vi "_createKafkaEvents.vi"(0 "Payload":string[](array[string]), 3 "error in (no error)":errorcluster, 4 "Debug":bool) -> (7 "Kafka Events":T1[](array[typedef]), 10 "error out":errorcluster)   [LabVIEW 2019]
uses:
  KafkaLVLib/API/KafkaConsumerEvent.ctl
  1f099e04-d0a3-4231-929c-9bf0d6f2adbc.vi
  <vilib>/JDP Science/JSONtext/String Subset.vi
  <vilib>/JDP Science/JSONtext/Parsing/Parse Full Path or Item Name.vi
  <vilib>/JDP Science/JSONtext/Next JSON Value.vi
  <vilib>/JDP Science/JSONtext/support/Error Cluster From Code.vi
  <vilib>/JDP Science/JSONtext/Offset/Find Item Locations by Path.vi
  <vilib>/JDP Science/JSONtext/JSON text to Variant.vi
  <vilib>/JDP Science/JSONtext/JSONtext.lvlib
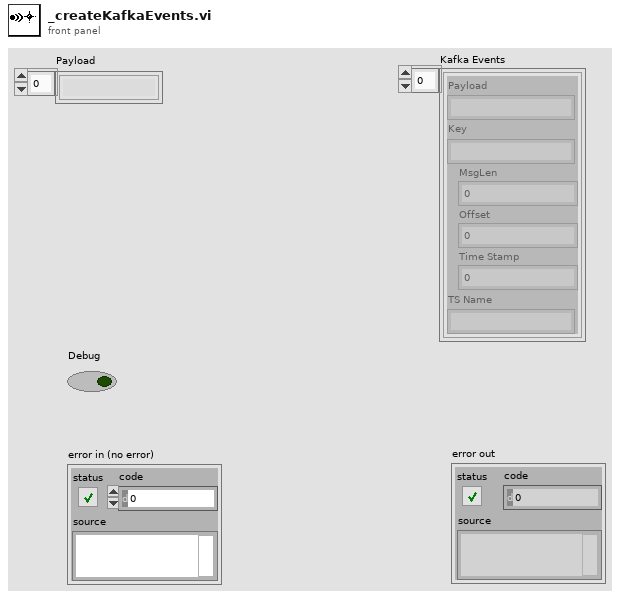
[diagram p1: front panel]
types:
  T1 = typedef "KafkaConsumerEvent.ctl" = cluster{"Payload":string, "Key":string, "MsgLen":u64, "Offset":i64, "Time Stamp":i64, "TS Name":string}
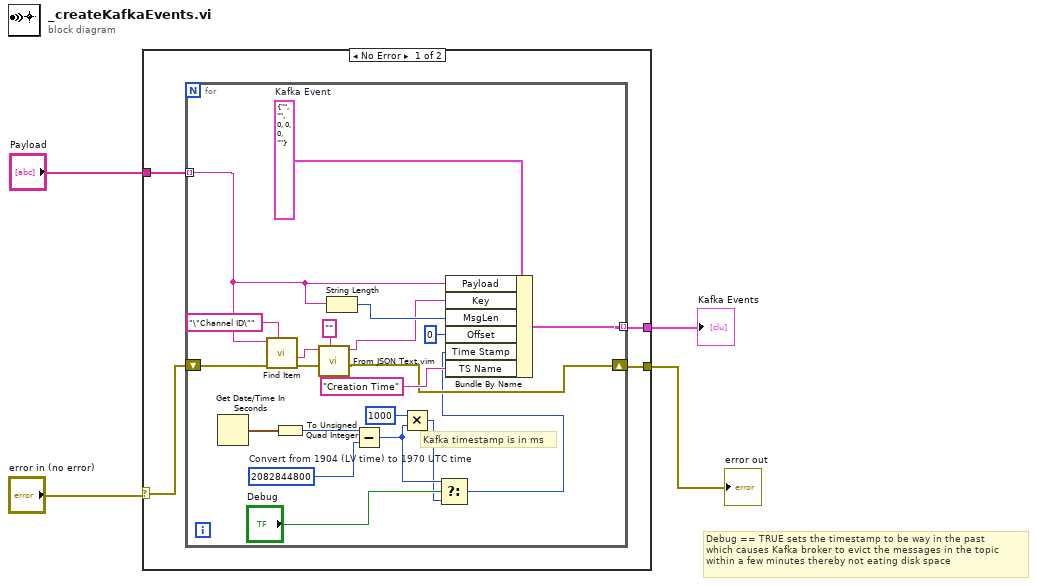
[diagram p0: block diagram]
diagram:
  # "Debug == TRUE sets the timestamp to be way in the past\nwhich causes Kafka broker to evict the messages in the topic \nwithin a few minutes thereby not eating disk space"
  n1 = case shown="No Error" "error in (no error)" {
    selector: "error in (no error)" -> [w7 w30]
    tunnel: "Payload" -> [w8 _]
    tunnel: [w6 w30] -> w2
    tunnel: [w5 _] -> w1
    frame No Error {
      n2 = for {
        tunnel: w8 -> [w26] mode=indexing
        shift-right: [w14] -> w6
        shift-left: w7 -> [w27]
        tunnel: [w19] -> w5 mode=indexing
        w22 = u64 2082844800  # Convert from 1904 (LV time) to 1970 UTC time
        w29 = T1 {"Payload"="", "Key"="", "MsgLen"=0, "Offset"=0, "Time Stamp"=0, "TS Name"=""}  # Kafka Event
        # "Kafka timestamp is in ms"
        n3 = Get Date/Time In Seconds() -> (seconds since 1Jan1904=w24:timestamp)
        n4 = call <vilib>:"Find Item.vi"("$Path or Item Name"="\"Channel ID\"", "error in (no error)"=w27, "JSON"=w26) -> ("error out"=w21:errorcluster, "<JSON>"=w17:string)  [unwired: 5 in, 2 out]
        n5 = To Unsigned Quad Integer(1:w24) -> (0:w23:u64)
        n6 = call "From JSON Text.vim"("Data Type and Default Value"="", "error in (no error)"=w21, "JSON"=w17) -> ("error out"=w14:errorcluster, "Data out"=w15:string)  [unwired: 7 in]
        n7 = String Length(string=w26) -> (length=w25:i32)
        n8 = Subtract(x=w23, y=w22) -> (x-y=w11:u64)
        n9 = Multiply(x=u64 1000, y=w11) -> (x*y=w10:u64)
        n10 = Select(t=w11, s="Debug", f=w10) -> (s? t:f=w9:u64)
        n11 = Bundle By Name(cluster=w29, "Payload"=w26, "Key"=w15, "MsgLen"=w25, "Offset"=i64 0, "Time Stamp"=w9, "TS Name"="Creation Time") -> (w19:T1)
      }
    }
    frame Error {
    }
  }
  "error out" <- w2
  "Kafka Events" <- w1
